vi "Determine Clicked Array Element Index - Calculate Scrollbar Edges.vi"(0 "Array Reference":refnum<vi>, 2 "Minimal Array Properties.Bounds":T2, 3 "Minimal Array Properties.Position":T1, 5 "error in (no error)":errorcluster, 6 "Select Item":T3(ring)) -> (14 "dup Array Reference":refnum<vi>, 16 "Minimum Scrollbar Edge":i32, 17 "Maximum Scrollbar Edge":i32, 19 "error out":errorcluster)   [LabVIEW 2011]
doc: "Determine Clicked Array Element Index - Calculate Scrollbar Edges.vi\n\nDescription:\nThis VI calculates the location of the edges of either the vertical or horizontal scrollbar.\n\nInputs:\nArray Reference - Reference to the array to operate on.\n\nMinimal Array Property.Bounds - Bounds property when the scrollbars, index display, label and caption are hidden.\n\nMinimal Array Property.Position - Position property when the scrollbars, index display, label and caption are hidden.\n\nSelect Item - Specifies the item to operate on.\n\nerror in - Standard error cluster.\n\nOutputs:\ndup Array Reference - Dup reference to the array to operate on.\n\nMinimum Scrollbar Edge - The location of the top or left edge of the selected scrollbar.\n\nMaximum Scrollbar Edge - The location of the bottom or richt edge of the selected scrollbar.\n\nerror out - standard error cluster.\n\nDeveloped By:\nMark.ridgley\nMark.Ridgley_LabVIEW.Developer@comcast.net"
uses:
  <vilib>/Utility/miscctls.llb/LVBoundsTypeDef.ctl
  <vilib>/Utility/miscctls.llb/LVPositionTypeDef.ctl
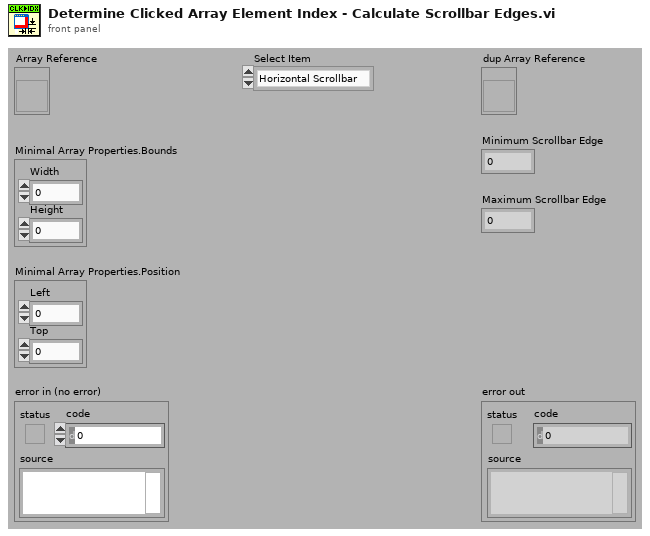
[diagram p1: front panel]
types:
  T1 = typedef "LVPositionTypeDef.ctl" = cluster{"Left":i32, "Top":i32}
  T2 = typedef "LVBoundsTypeDef.ctl" = cluster{"Width":u32, "Height":u32}
  T3 = enum16{"Horizontal Scrollbar", "Vertical Scrollbar"}
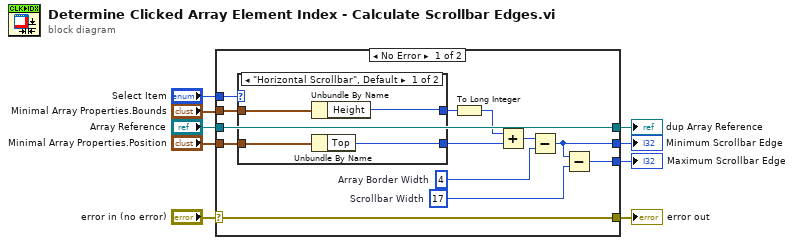
[diagram p0: block diagram]
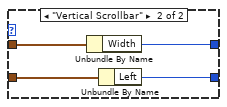
[diagram p2: hidden frame]
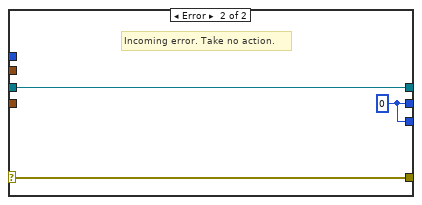
[diagram p3: hidden frame]
diagram:
  n1 = case shown="No Error" "error in (no error)" {
    selector: "error in (no error)" -> [w22 w32]
    tunnel: [w12 w31] -> w9
    tunnel: [w10 w31] -> w8
    tunnel: "Array Reference" -> [w21 w33]
    tunnel: [w22 w32] -> w6
    tunnel: [w21 w33] -> w4
    tunnel: "Minimal Array Properties.Bounds" -> [w20 _]
    tunnel: "Minimal Array Properties.Position" -> [w19 _]
    tunnel: "Select Item" -> [w18 _]
    frame No Error {
      w16 = 17  # Scrollbar Width
      w15 = 4  # Array Border Width
      n2 = case shown="\"Horizontal Scrollbar\", Default" w18 {
        tunnel: [w23 w27] -> w11
        tunnel: w20 -> [w26 w30]
        tunnel: w19 -> [w25 w29]
        tunnel: [w24 w28] -> w13
        frame "Horizontal Scrollbar", Default {
          n3 = Unbundle By Name(w26) -> ("Height"=w24:u32)
          n4 = Unbundle By Name(w25) -> ("Top"=w23:i32)
        }
        frame "Vertical Scrollbar" {
          n5 = Unbundle By Name(w30) -> ("Width"=w28:u32)
          n6 = Unbundle By Name(w29) -> ("Left"=w27:i32)
        }
      }
      n7 = To Long Integer(number=w13) -> (32bit integer=w17:i32)
      n8 = Add(x=w17, y=w11) -> (x+y=w14:i32)
      n9 = Subtract(x=w14, y=w15) -> (x-y=w10:i32)
      n10 = Subtract(x=w10, y=w16) -> (x-y=w12:i32)
    }
    frame Error {
      w31 = 0
      # "Incoming error. Take no action."
    }
  }
  "Maximum Scrollbar Edge" <- w9
  "Minimum Scrollbar Edge" <- w8
  "dup Array Reference" <- w4
  "error out" <- w6
